vi "Red Pitaya Lockin.vi"(8 "Error In":errorcluster, 10 "Server port":u16=1002, 11 "Server address":string="192.168.1.100") -> (0 "Error Out":errorcluster)   [LabVIEW 2016]
uses:
  Mode.ctl
  Red Pitaya Parameters.ctl
  RP Command.ctl
  RP Write Command TCP.vi
  RP Read Status TCP.vi
  RP Read Temperature TCP.vi
  RP Read Subset TCP.vi
panel:
  out "FIFO counter":u32
  in  "Read FIFO":bool
  out "Waveform Chart 3":i32[](graph)
  out "Waveform Chart 2":i32[](graph)
  out "Waveform Chart":i32[](graph)
  out "last update, ms":i32
  in  "Controls":enum32{"Basic", "Advanced"}(tab)
  in  "Parameters":T1={"Ranges"=[20.0, 20.0], "Output frequency 1"=50000.0, "Output frequency 2"=50000.0, "Pre-trigger samples"=-100000, "Post-trigger samples"=67108864, "Desimation rate"=8192, "Delayed start"=571428} {"Delayed start" format="0x%x (%d)"; "Post-trigger samples" format="0x%x (%d)"; "Pre-trigger samples" format="0x%x (%d)"; "Output frequency 2" format="%#_6p"; "Output frequency 1" format="%#_6p"; "Ranges" format="%#_12p"}
  out "CPU Temperature":dbl(slide)=48.847186279148 scale=0.0..100.0
  in  "Trigger pos acuracy":i32=2
  in  "Signal bits":i32=14
  in  "Read Temperature":bool=TRUE
  in  "Read trigger":bool=TRUE
  in  "Start server":bool
  in  "FPGA Logic":enum16{"Digitizer", "Fast Digitizer"}(ring)
  in  "Auto-save file":bool=TRUE
  in  "Samples to read":u64=67108864 format="0x%x (%d)"
  in  "Record":bool
  out "Server  output":string
  out "Temperature Chart":dbl(graph)=48.847186279148
  out "bytes written":i32=8
  in  "Status":bool
  out "Status response":u32=1
  out "element":u32
  in  "Status offset":u64=8 format="%x"
  out "Record start pos":u32=1
  out "x-y":u32=4294967295
  out "Phase increment 2":u64=1717987
  out "Phase increment 1":u64=1717987
  in  "Process Stop Button":bool
  in  "Read All":bool
  in  "Read subset":bool
  out "Data File  Path":path
  out "Trigger state":bool
  in  "Trigger":bool
  in  "Arm":bool
  out "Phase  Graph":u32[](graph)
  in  "Mode":T2=enum."Digitizer"
  out "Waveform Graph":sgl[][](graph)
  in  "Stop Server":bool
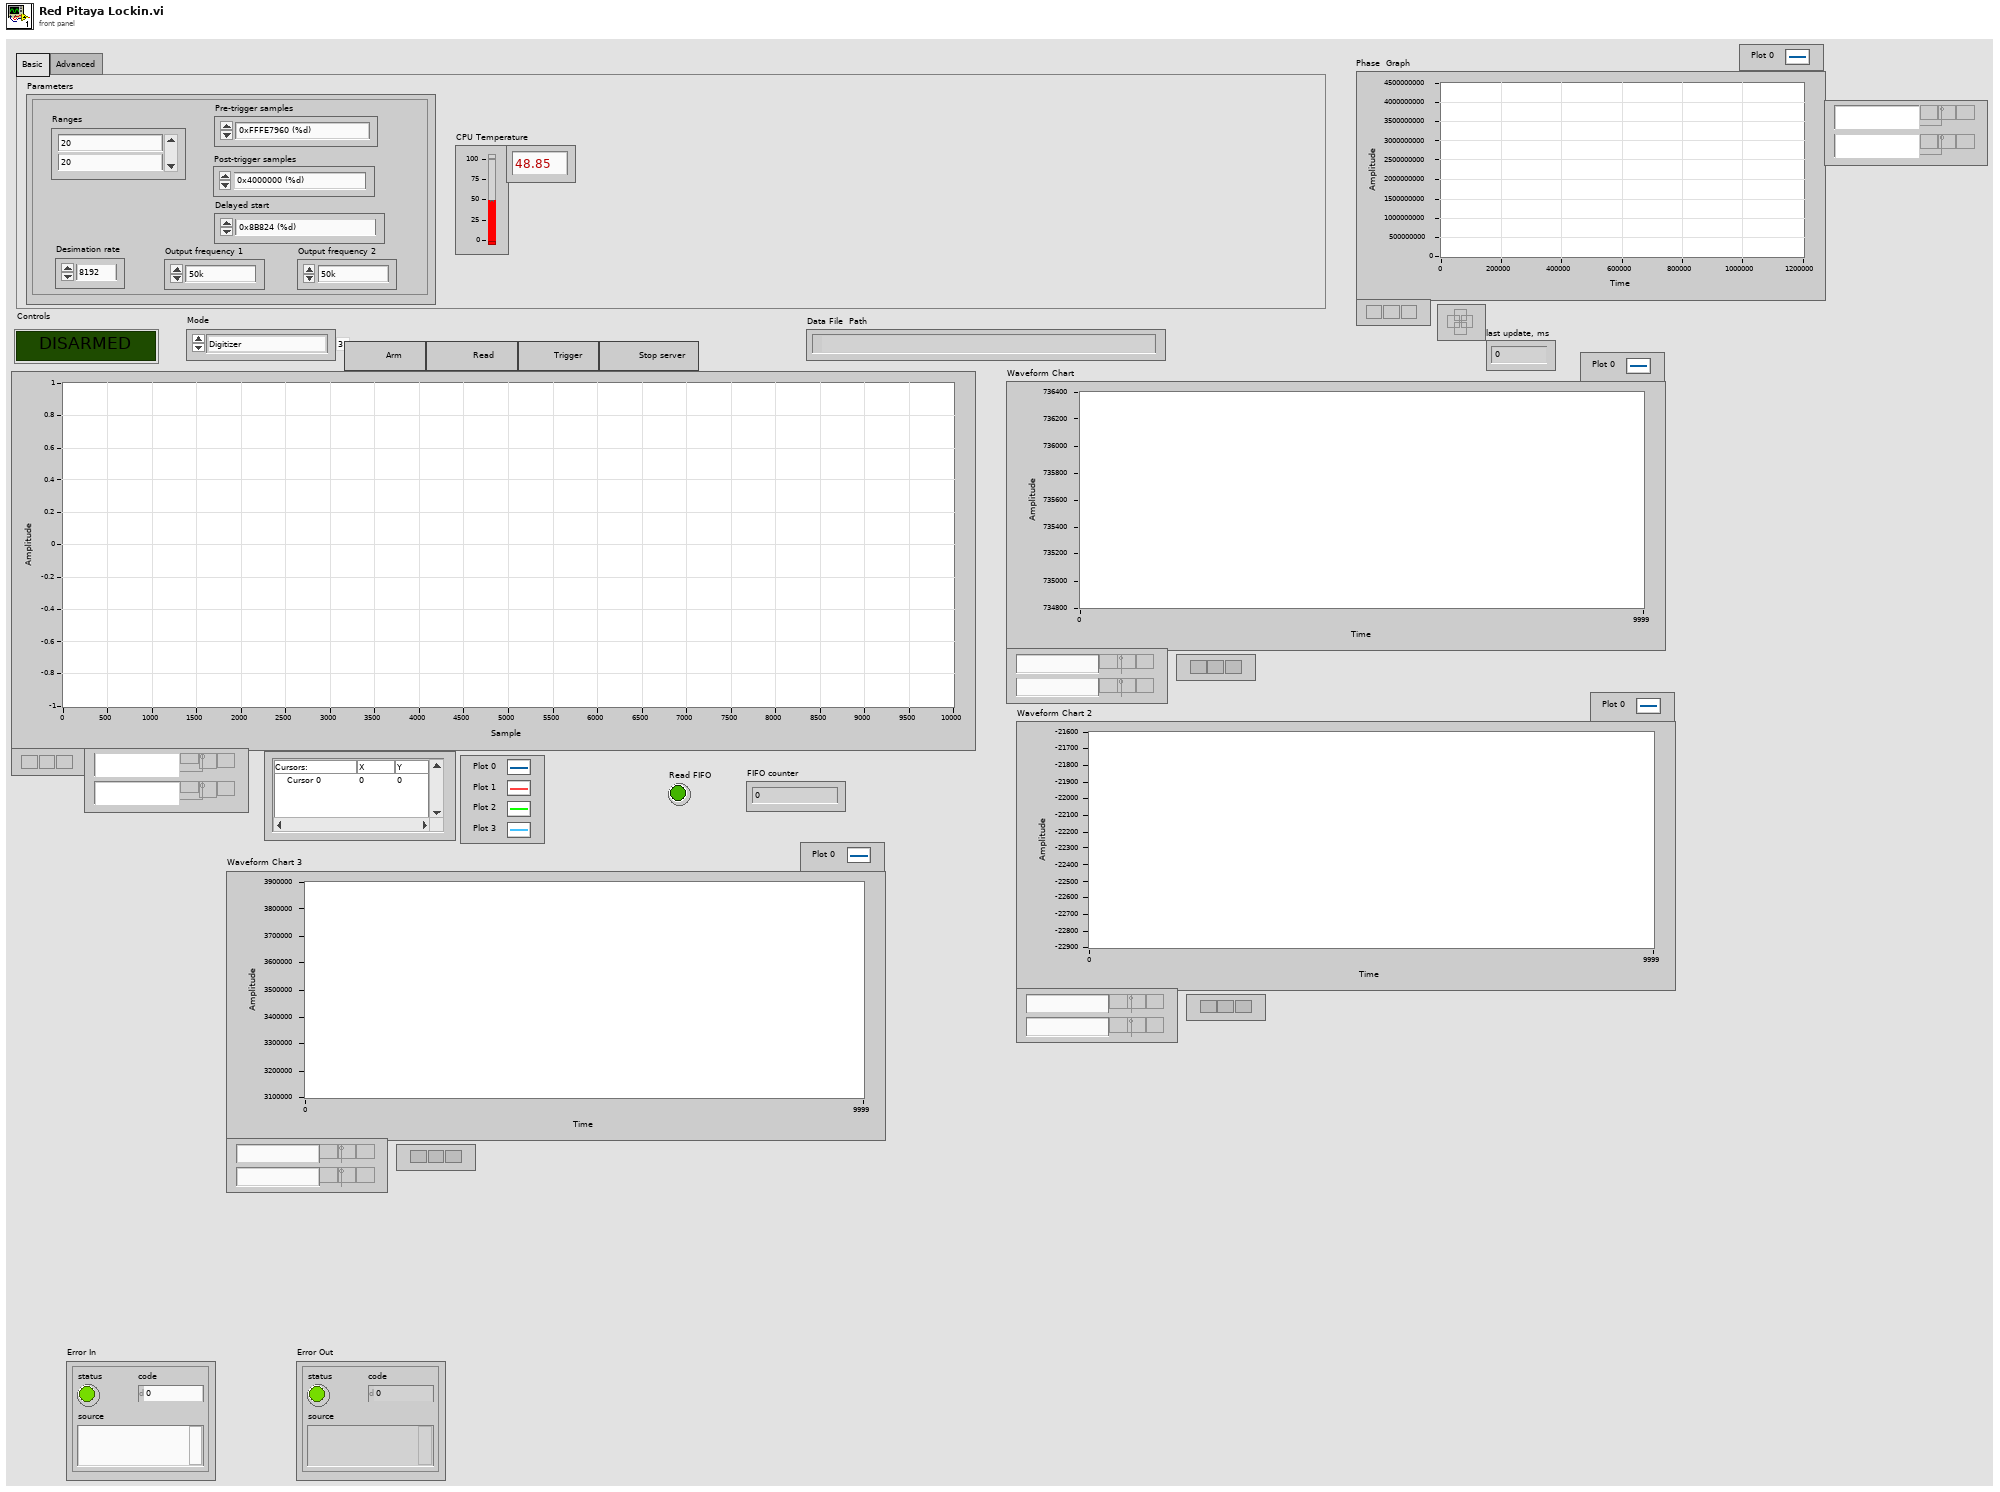
[diagram p1: front panel]
types:
  T1 = typedef "Red Pitaya Parameters.ctl" = cluster{"Ranges":dbl[], "Output frequency 1":dbl, "Output frequency 2":dbl, "Pre-trigger samples":i32, "Post-trigger samples":u64, "Desimation rate":u64, "Delayed start":u64}
  T2 = typedef "Mode.ctl" = enum16{"Filter", "Lockin test", "Snapshot test", "Digitizer", "Current-Voltage"}
  T3 = typedef "RP Command.ctl" = enum16{"Reset", "Read IDN", "Stop server", "Get status", "Get temperature", "Connect client", "Arm", "Software trigger", "Get whole buffer", "Get chunk", "System call", "Get config", "Set config", "Recieve data", "Recieve Calibartion", "Transmit data"}
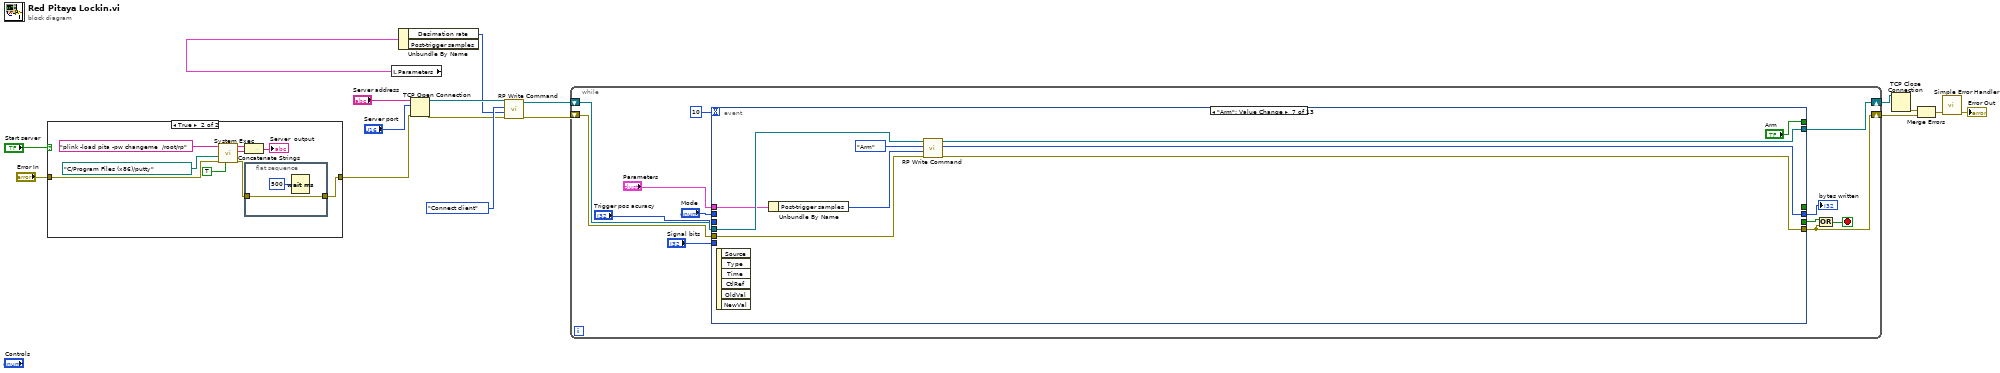
[diagram p0: block diagram]
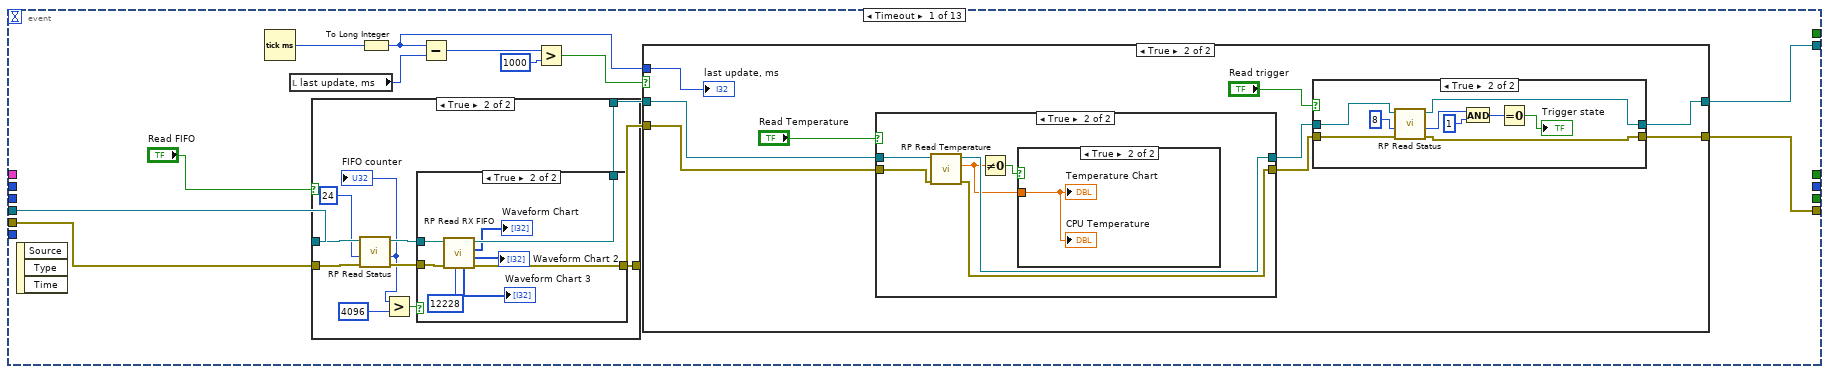
[diagram p3: hidden frame]
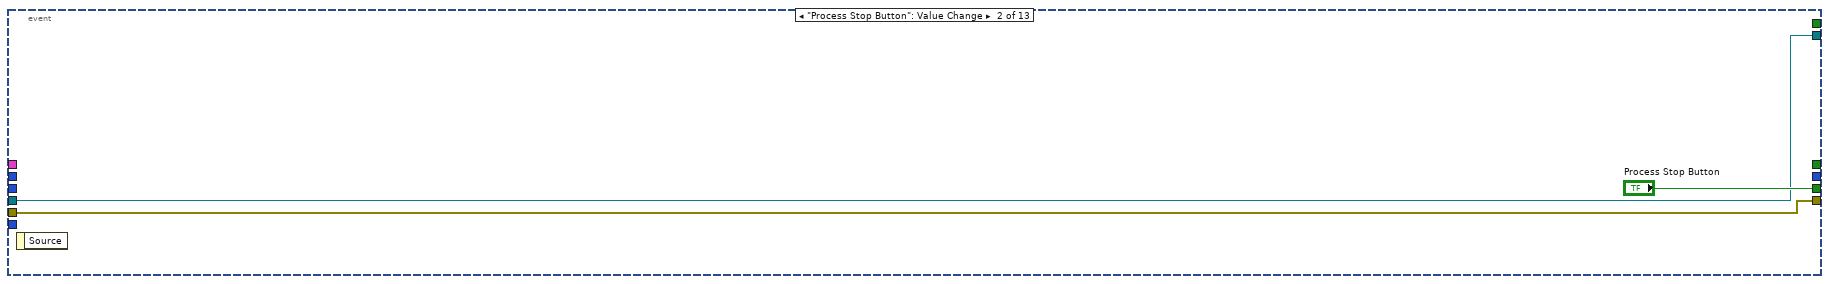
[diagram p10: hidden frame]
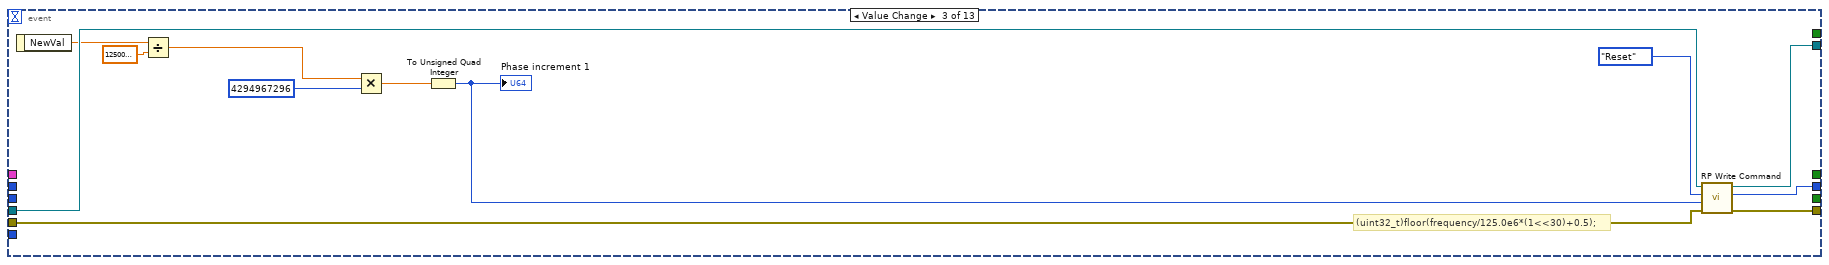
[diagram p11: hidden frame]
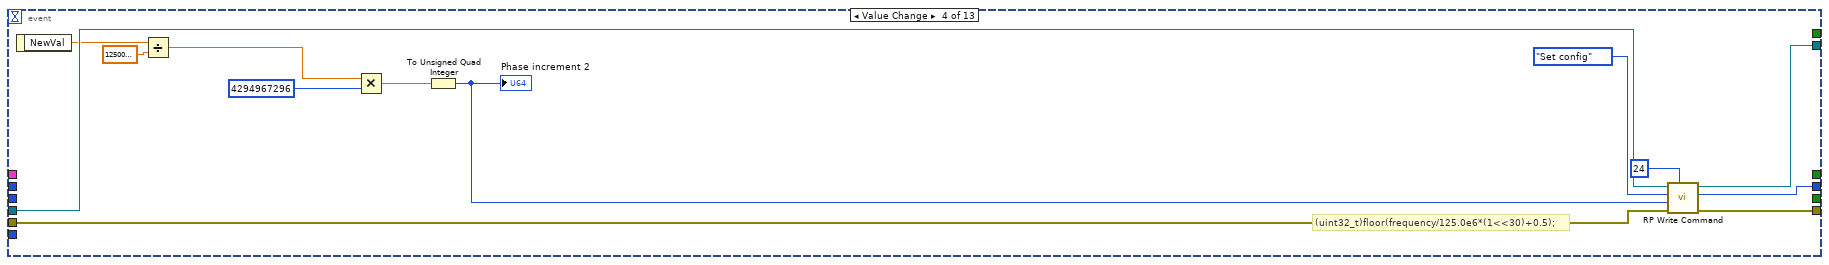
[diagram p12: hidden frame]
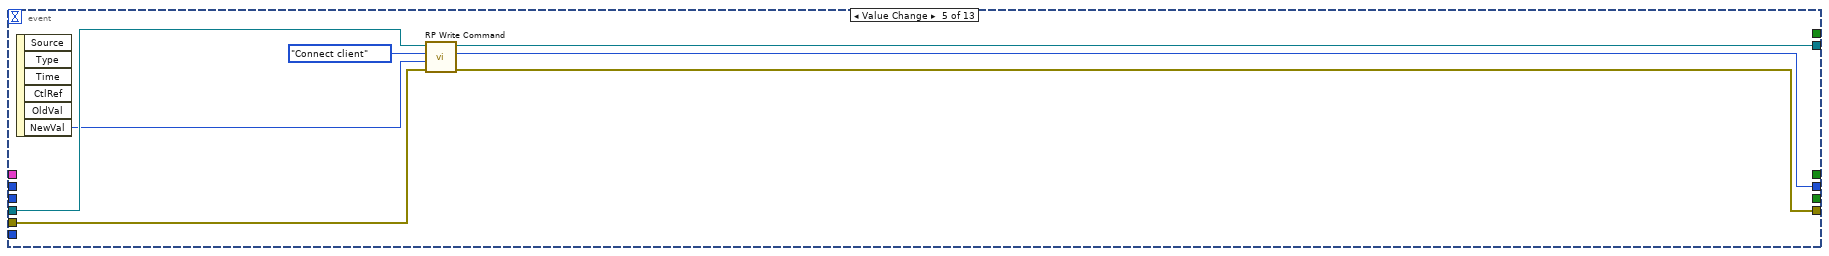
[diagram p13: hidden frame]
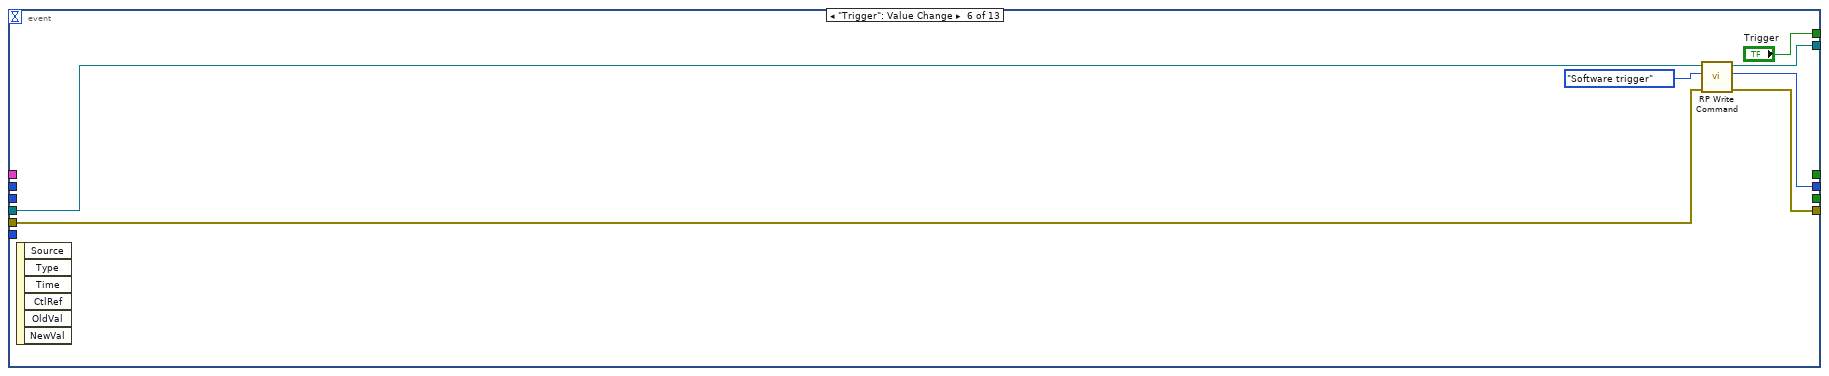
[diagram p14: hidden frame]
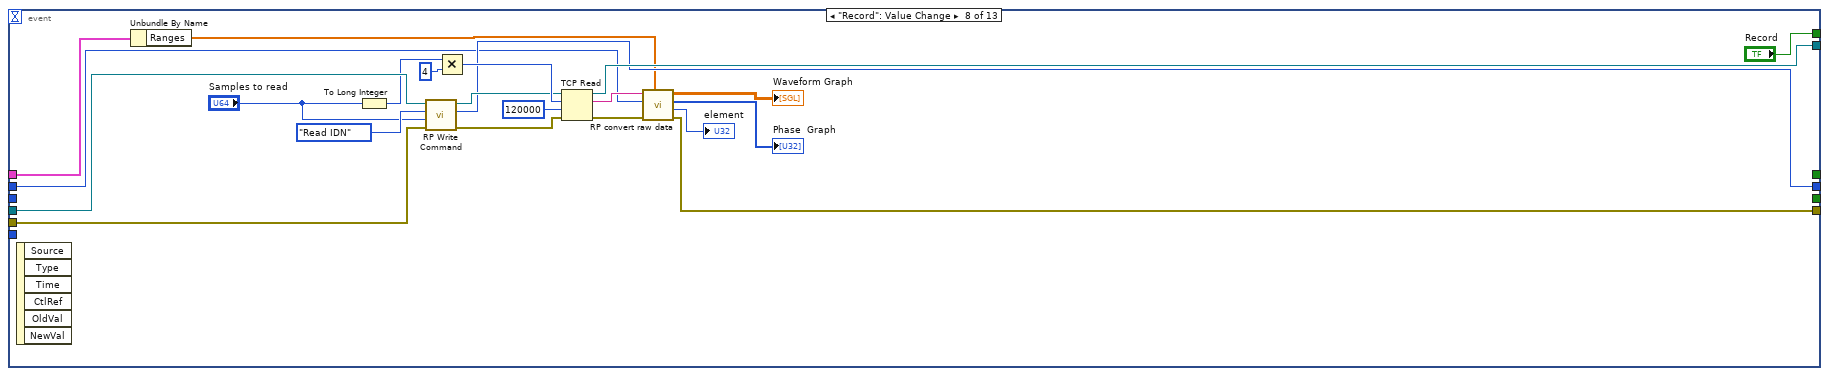
[diagram p15: hidden frame]
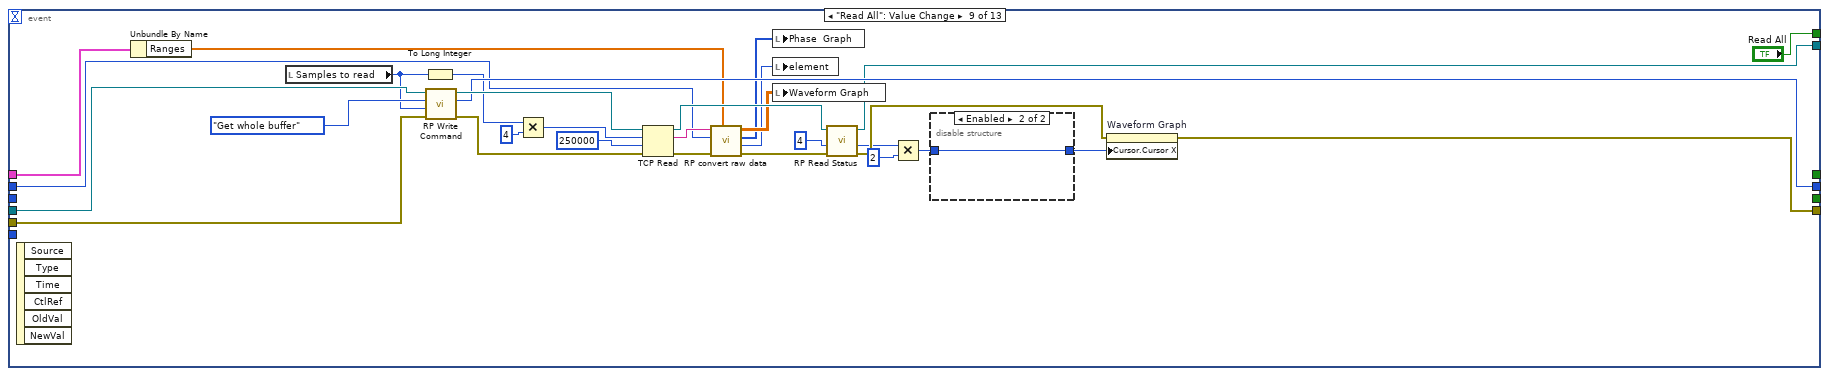
[diagram p16: hidden frame]
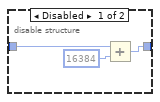
[diagram p17: hidden frame]
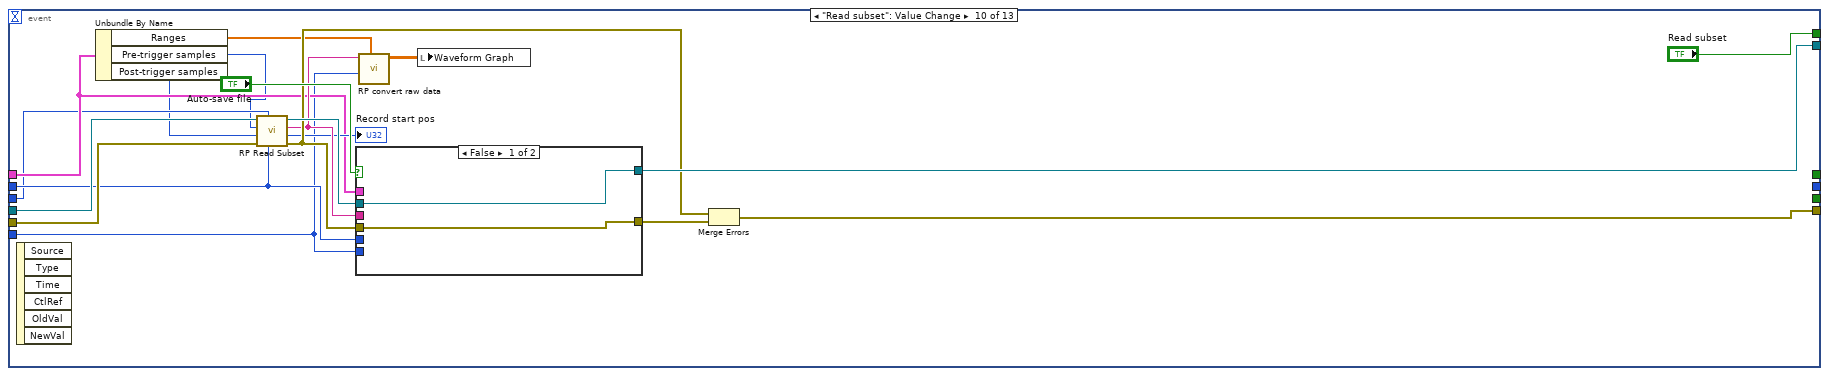
[diagram p18: hidden frame]
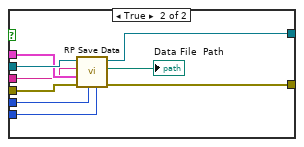
[diagram p19: hidden frame]
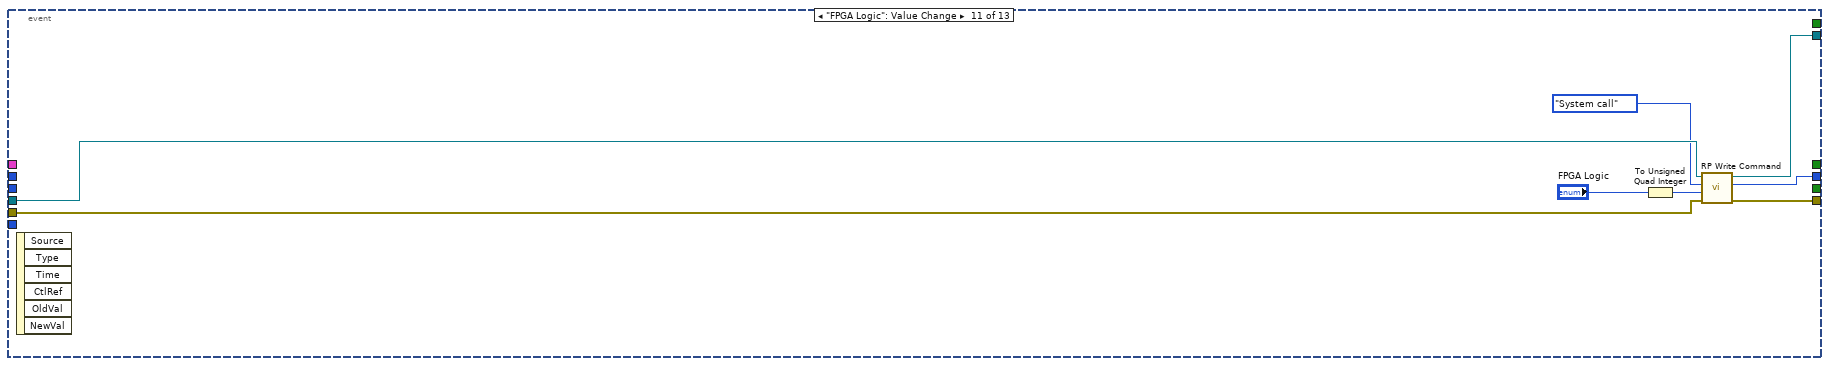
[diagram p20: hidden frame]
diagram:
  n1 = case shown="True" "Start server" {
    tunnel: [w18 w19] -> w9
    tunnel: "Error In" -> [w18 w21]
    frame False {
    }
    frame True {
      n2 = call <vilib>:"System Exec.vi"("run minimized? (F)"=TRUE, "error in (no error)"=w21, "working directory"=path "C:/Program Files (x86)/putty", "command line"="plink -load pita -pw changeme  /root/rp") -> ("error out"=w20:errorcluster, "standard error"=w23:string, "standard output"=w27:string)  [unwired: 4 in, 1 out]
      n3 = Concatenate Strings(w27, w23) -> (→"Server  output":string)
      n4 = flat-sequence {
        tunnel: w20 -> [w29]
        tunnel: [w29] -> w19
        frame #0 {
          n5 = Wait (ms)(milliseconds to wait=u32 500) -> ()  [unwired: 1 out]
        }
      }
    }
  }
  n6 = local read "Parameters"() -> (w6:T1)
  n7 = Unbundle By Name(w6) -> ("Desimation rate"=w3:u64)  [unwired: 1 out]
  n8 = TCP Open Connection(address="Server address", remote port or service name="Server port", error in (no error)=w9) -> (connection ID=w5:refnum<k5>, error out=w2:errorcluster)  [unwired: 2 in]
  n9 = call-poly "RP Write Command.vi"("Error In"=w2, "Command payload"=w3, "Command number"=RP_Command."Connect client", "connection ID"=w5) -> ("Error Out"=w1:errorcluster, "connection ID out"=w4:refnum<k5>)  [unwired: 5 in, 1 out]
  n10 = while {
    shift-right: [w39] -> w13
    shift-left: w4 -> [w40]
    shift-right: [w37] -> w12
    shift-left: w1 -> [w41]
    stop <- w35 stop-if-true
    n11 = event shown="[6] \"Arm\": Value Change" {
      selector: _ -> [_ _ _ _ _ _ _ _ _ _ _ _ _]
      dyn-events: _ -> [_ _ _ _ _ _ _ _ _ _ _ _ _]
      timeout: 10 -> [_ _ _ _ _ _ _ _ _ _ _ _ _]
      tunnel: w41 -> [w44 w109 w118 w131 w142 w149 w158 w173 w205 w227 w252 w259 w265]
      tunnel: w40 -> [w46 w108 w117 w130 w141 w148 w157 w176 w208 w226 w251 w257 w261]
      tunnel: [w54 w109 w113 w126 w138 w145 w154 w164 w202 w231 w247 w256 w264] -> w37
      tunnel: [w53 w108 w114 w127 w139 w146 w155 w178 w198 w228 w246 w255 w262] -> w39
      tunnel: [_ "Process Stop Button" _ _ _ _ _ _ _ _ _ "Stop Server" _] -> w36
      tunnel: [_ _ _ _ _ _ _ _ _ _ _ _ "Status"] -> _
      tunnel: [_ _ w112 w125 w137 w144 w153 w171 w203 _ w245 w254 _] -> w38
      tunnel: [_ _ _ _ _ "Trigger" "Arm" "Record" "Read All" "Read subset" _ _ _] -> _
      tunnel: "Mode" -> [_ _ _ _ _ _ _ w161 w183 w222 _ _ _]
      tunnel: "Parameters" -> [_ _ _ _ _ _ w151 w160 w182 w220 _ _ _]
      tunnel: "Signal bits" -> [_ _ _ _ _ _ _ _ _ w217 _ _ _]
      tunnel: "Trigger pos acuracy" -> [_ _ _ _ _ _ _ _ _ w218 _ _ _]
      event Timeout {
        n12 = event-data() -> ()  [unwired: 1 in, 3 out]
        n13 = Tick Count (ms)() -> (millisecond timer value=w52:u32)
        n14 = local read "last update, ms"() -> (w51:i32)
        n15 = case shown="True" "Read FIFO" {
          tunnel: w46 -> [w55 w61]
          tunnel: [w55 w66] -> w45
          tunnel: w44 -> [w56 w64]
          tunnel: [w56 w65] -> w43
          frame False {
          }
          frame True {
            n16 = call-poly "RP Read Status.vi"("Error In"=w64, "Status offset"=u64 24, "connection ID"=w61) -> ("Error Out"=w63:errorcluster, "Status response"=w59:u32, "connection ID out"=w62:refnum<k5>)  [unwired: 6 in]
            "FIFO counter" <- w59
            n17 = Greater?(x=w59, y=u32 4096) -> (0:w57:bool)
            n18 = case shown="True" w57 {
              tunnel: w62 -> [w67 w76]
              tunnel: [w67 w75] -> w66
              tunnel: [w68 w74] -> w65
              tunnel: w63 -> [w68 w70]
              frame False {
              }
              frame True {
                n19 = call "RP Read RX FIFO.vi"("FIFO Bytes per read"=12228, "Error In"=w70, "connection ID"=w76) -> ("Error Out"=w74:errorcluster, "Y"=→"Waveform Chart 2":i32[], "X"=→"Waveform Chart":i32[], "connection ID out"=w75:refnum<k5>, "F"=→"Waveform Chart 3":i32[])  [unwired: 4 in]
              }
            }
          }
        }
        n20 = To Long Integer(number=w52) -> (32bit integer=w47:i32)
        n21 = Subtract(x=w47, y=w51) -> (x-y=w50:i32)
        n22 = Greater?(x=w50, y=1000) -> (0:w48:bool)
        n23 = case shown="True" w48 {
          tunnel: w45 -> [w77 w86]
          tunnel: w43 -> [w78 w85]
          tunnel: [w78 w81] -> w54
          tunnel: [w77 w80] -> w53
          tunnel: w47 -> [_ w79]
          frame False {
          }
          frame True {
            n24 = case shown="True" "Read Temperature" {
              tunnel: w86 -> [w100 w105]
              tunnel: w85 -> [w99 w101]
              tunnel: [w100 w104] -> w83
              tunnel: [w99 w102] -> w82
              frame False {
              }
              frame True {
                n25 = call-poly "RP Read Temperature.vi"("Error In"=w101, "connection ID"=w105) -> ("error out"=w102:errorcluster, "Thermometer"=w103:dbl, "connection ID out"=w104:refnum<k5>)  [unwired: 7 in]
                n26 = Not Equal To 0?(x=w103) -> (x != 0?=w106:bool)
                n27 = case shown="True" w106 {
                  tunnel: w103 -> [_ w107]
                  frame False {
                  }
                  frame True {
                    "CPU Temperature" <- w107
                    "Temperature Chart" <- w107
                  }
                }
              }
            }
            n28 = case shown="True" "Read trigger" {
              tunnel: w83 -> [w88 w97]
              tunnel: w82 -> [w89 w98]
              tunnel: [w89 w93] -> w81
              tunnel: [w88 w90] -> w80
              frame False {
              }
              frame True {
                n29 = call-poly "RP Read Status.vi"("Error In"=w98, "Status offset"=u64 8, "connection ID"=w97) -> ("Error Out"=w93:errorcluster, "Status response"=w95:u32, "connection ID out"=w90:refnum<k5>)  [unwired: 6 in]
                n30 = And(x=w95, y=u32 1) -> (x .and. y?=w92:u32)
                n31 = Equal To 0?(x=w92) -> (x = 0?=→"Trigger state":bool)
              }
            }
            "last update, ms" <- w79
          }
        }
      }
      event "Process Stop Button": Value Change {
        n32 = event-data() -> ()  [unwired: 1 in, 1 out]
      }
      event Value Change {
        # "(uint32_t)floor(frequency/125.0e6*(1<<30)+0.5);"
        n33 = event-data() -> ("NewVal"=w111:dbl)  [unwired: 1 in]
        n34 = Divide(x=w111, y=125000000.0) -> (x/y=w120:dbl)
        n35 = Multiply(x=w120, y=i64 4294967296) -> (x*y=w119:dbl)
        n36 = To Unsigned Quad Integer(1:w119) -> (0:w115:u64)
        "Phase increment 1" <- w115
        n37 = call-poly "RP Write Command.vi"("Error In"=w118, "Command payload"=w115, "Command number"=RP_Command."Reset", "connection ID"=w117) -> ("Error Out"=w113:errorcluster, "bytes written"=w112:i32, "connection ID out"=w114:refnum<k5>)  [unwired: 5 in]
      }
      event Value Change {
        # "(uint32_t)floor(frequency/125.0e6*(1<<30)+0.5);"
        n38 = event-data() -> ("NewVal"=w123:dbl)  [unwired: 1 in]
        n39 = Divide(x=w123, y=125000000.0) -> (x/y=w133:dbl)
        n40 = Multiply(x=w133, y=i64 4294967296) -> (x*y=w132:dbl)
        n41 = To Unsigned Quad Integer(1:w132) -> (0:w128:u64)
        "Phase increment 2" <- w128
        n42 = call-poly "RP Write Command.vi"("Config offset"=u64 24, "Error In"=w131, "Command payload"=w128, "Command number"=RP_Command."Set config", "connection ID"=w130) -> ("Error Out"=w126:errorcluster, "bytes written"=w125:i32, "connection ID out"=w127:refnum<k5>)  [unwired: 4 in]
      }
      event Value Change {
        n43 = event-data() -> ("NewVal"=w136:u64)  [unwired: 1 in, 5 out]
        n44 = call-poly "RP Write Command.vi"("Error In"=w142, "Command payload"=w136, "Command number"=RP_Command."Connect client", "connection ID"=w141) -> ("Error Out"=w138:errorcluster, "bytes written"=w137:i32, "connection ID out"=w139:refnum<k5>)  [unwired: 5 in]
      }
      event "Trigger": Value Change {
        n45 = event-data() -> ()  [unwired: 1 in, 6 out]
        n46 = call-poly "RP Write Command.vi"("Error In"=w149, "Command number"=RP_Command."Software trigger", "connection ID"=w148) -> ("Error Out"=w145:errorcluster, "bytes written"=w144:i32, "connection ID out"=w146:refnum<k5>)  [unwired: 6 in]
      }
      event "Arm": Value Change {
        n47 = event-data() -> ()  [unwired: 1 in, 6 out]
        n48 = Unbundle By Name(w151) -> ("Post-trigger samples"=w150:u64)
        n49 = call-poly "RP Write Command.vi"("Error In"=w158, "Command payload"=w150, "Command number"=RP_Command."Arm", "connection ID"=w157) -> ("Error Out"=w154:errorcluster, "bytes written"=w153:i32, "connection ID out"=w155:refnum<k5>)  [unwired: 5 in]
      }
      event "Record": Value Change {
        n50 = event-data() -> ()  [unwired: 1 in, 6 out]
        n51 = Unbundle By Name(w160) -> ("Ranges"=w159:dbl[])
        n52 = To Long Integer(number="Samples to read") -> (32bit integer=w170:i32)
        n53 = call-poly "RP Write Command.vi"("Error In"=w173, "Command payload"="Samples to read", "Command number"=RP_Command."Read IDN", "connection ID"=w176) -> ("Error Out"=w172:errorcluster, "bytes written"=w171:i32, "connection ID out"=w174:refnum<k5>)  [unwired: 5 in]
        n54 = Multiply(x=w170, y=4) -> (x*y=w177:i32)
        n55 = TCP Read(connection ID=w174, bytes to read=w177, error in (no error)=w172, 9:120000 ("timeout ms (25000)")) -> (connection ID out=w178:refnum<k5>, data out=w167:string, error out=w165:errorcluster)  [unwired: 1 in]
        n56 = call "RP convert raw data.vi"("Max Volts"=w159, "Error In"=w165, "Format"=w161, "data stream"=w167) -> ("Error Out"=w164:errorcluster, "element"=→"element":u32, "phase out"=→"Phase  Graph":u32[], "data out"=→"Waveform Graph":sgl[][])  [unwired: 4 in]
      }
      event "Read All": Value Change {
        n57 = event-data() -> ()  [unwired: 1 in, 6 out]
        n58 = Unbundle By Name(w182) -> ("Ranges"=w181:dbl[])
        n59 = local read "Samples to read"() -> (w197:u64)
        n60 = To Long Integer(number=w197) -> (32bit integer=w200:i32)
        n61 = call-poly "RP Write Command.vi"("Error In"=w205, "Command payload"=w197, "Command number"=RP_Command."Get whole buffer", "connection ID"=w208) -> ("Error Out"=w204:errorcluster, "bytes written"=w203:i32, "connection ID out"=w206:refnum<k5>)  [unwired: 5 in]
        n62 = Multiply(x=w200, y=4) -> (x*y=w209:i32)
        n63 = TCP Read(connection ID=w206, bytes to read=w209, error in (no error)=w204, 9:250000 ("timeout ms (25000)")) -> (connection ID out=w199:refnum<k5>, data out=w195:string, error out=w185:errorcluster)  [unwired: 1 in]
        n64 = call "RP convert raw data.vi"("Max Volts"=w181, "Error In"=w185, "Format"=w183, "data stream"=w195) -> ("Error Out"=w184:errorcluster, "element"=w192:u32, "phase out"=w193:u32[], "data out"=w194:sgl[][])  [unwired: 4 in]
        n65 = local write "Phase  Graph"(w193) -> ()
        n66 = local write "element"(w192) -> ()
        n67 = local write "Waveform Graph"(w194) -> ()
        n68 = call-poly "RP Read Status.vi"("Error In"=w184, "Status offset"=u64 4, "connection ID"=w199) -> ("Error Out"=w190:errorcluster, "Status response"=w189:u32, "connection ID out"=w198:refnum<k5>)  [unwired: 6 in]
        n69 = Multiply(x=w189, y=u32 2) -> (x*y=w187:u32)
        n70 = disable-structure shown="Enabled" {
          disable-tunnel: w187 -> [w213 w214]
          disable-tunnel: [w211 w214] -> w186
          frame Disabled {
            n71 = Add(x=w213, y=16384) -> (x+y=w211:u32)
          }
          frame Enabled {
          }
        }
        n72 = property on="Waveform Graph" class="WFGraph (strict)"(error in=w190, "Cursor.Cursor X"=w186) -> (error out=w202:errorcluster)  [unwired: 1 in, 1 out]
      }
      event "Read subset": Value Change {
        n73 = event-data() -> ()  [unwired: 1 in, 6 out]
        n74 = Unbundle By Name(w220) -> ("Ranges"=w219:dbl[], "Pre-trigger samples"=w216:i32, "Post-trigger samples"=w215:u64)
        n75 = call-poly "RP Read Subset.vi"("Bytes per sample"=w222, "Samples per trigger increment"=w218, "Error In"=w227, "Post-trigger samples"=w215, "Pre-trigger samples"=w216, "connection ID"=w226) -> ("Error Out"=w224:errorcluster, "Record start pos"=→"Record start pos":u32, "Data stream"=w223:string, "connection ID out"=w225:refnum<k5>)  [unwired: 2 in]
        n76 = case shown="False" "Auto-save file" {
          tunnel: w224 -> [w235 w238]
          tunnel: w223 -> [_ w242]
          tunnel: [w235 w237] -> w230
          tunnel: w225 -> [w234 w244]
          tunnel: [w234 w240] -> w228
          tunnel: w220 -> [_ w243]
          tunnel: w222 -> [_ w241]
          tunnel: w217 -> [_ w236]
          frame False {
          }
          frame True {
            n77 = call "RP Save Data.vi"("Signal bits"=w236, "Mode"=w241, "Error In"=w238, "Parameters"=w243, "Data stream"=w242, "connection ID"=w244) -> ("Error Out"=w237:errorcluster, "Data File  Path"=→"Data File  Path":path, "connection ID out"=w240:refnum<k5>)  [unwired: 2 in, 1 out]
          }
        }
        n78 = call "RP convert raw data.vi"("Max Volts"=w219, "Signal bits"=w217, "data stream"=w223) -> ("data out"=w229:sgl[][])  [unwired: 5 in, 3 out]
        n79 = local write "Waveform Graph"(w229) -> ()
        n80 = Merge Errors(w224, w230) -> (w231:errorcluster)
      }
      event "FPGA Logic": Value Change {
        n81 = event-data() -> ()  [unwired: 1 in, 6 out]
        n82 = To Unsigned Quad Integer(1:"FPGA Logic") -> (0:w249:u64)
        n83 = call-poly "RP Write Command.vi"("Error In"=w252, "Command payload"=w249, "Command number"=RP_Command."System call", "connection ID"=w251) -> ("Error Out"=w247:errorcluster, "bytes written"=w245:i32, "connection ID out"=w246:refnum<k5>)  [unwired: 5 in]
      }
      event "Stop Server": Value Change {
        n84 = event-data() -> ()  [unwired: 1 in, 6 out]
        n85 = call-poly "RP Write Command.vi"("Error In"=w259, "Command number"=RP_Command."Stop server", "connection ID"=w257) -> ("Error Out"=w256:errorcluster, "bytes written"=w254:i32, "connection ID out"=w255:refnum<k5>)  [unwired: 6 in]
      }
      event "Status": Value Change {
        n86 = event-data() -> ()  [unwired: 1 in, 6 out]
        n87 = local read "element"() -> (w267:u32)
        n88 = call-poly "RP Read Status.vi"("Error In"=w265, "Status offset"="Status offset", "connection ID"=w261) -> ("Error Out"=w264:errorcluster, "Status response"=w263:u32, "connection ID out"=w262:refnum<k5>)  [unwired: 6 in]
        "Status response" <- w263
        n89 = Subtract(x=w267, y=w263) -> (x-y=→"x-y":u32)
      }
    }
    "bytes written" <- w38
    n90 = Or(x=w36, y=w37) -> (x .or. y?=w35:bool)
  }
  n91 = TCP Close Connection(connection ID=w13) -> (error out=w15:errorcluster)  [unwired: 2 in, 1 out]
  n92 = Merge Errors(w15, w12) -> (w14:errorcluster)
  n93 = call <vilib>:"Simple Error Handler.vi"("error in (no error)"=w14) -> ("error out"=→"Error Out":errorcluster)  [unwired: 4 in, 4 out]
